vi "example_vector_add_vectors.vi"() -> ()   [LabVIEW 2020]
uses:
  src/vectorstore/abstract_vector_base/abstract_vector_base.lvclass
  src/vectorstore/abstract_vector_base/vector.ctl
  src/models/llm_openai_embedding/llm_openai_embedding.lvclass
  D:/Personal/LabVIEW LLMs/src/models/abstract_llm_base/abstract_llm_base.lvclass
  src/vectorstore/vector_qdrant/vector_qdrant.lvclass
  D:/Personal/LabVIEW LLMs/src/vectorstore/abstract_vector_base/abstract_vector_base.lvclass
  src/models/message_text/message_text.lvclass
  D:/Personal/LabVIEW LLMs/src/models/abstract_message_base/abstract_message_base.lvclass
  src/models/message_vectors/message_vectors.lvclass
  src/models/message_text/create_text_message.vi
  src/models/llm_openai_embedding/Instantiate_llm_openai_embed.vi
  src/models/message_text/get_text_message_value.vi
  src/models/message_vectors/get_vector_message_value.vi
  src/utilities/env_variables/env_variables.lvlib
  src/models/abstract_llm_embedding/abstract_llm_embedding.lvclass
  D:/Personal/LabVIEW LLMs/src/models/message_text/message_text.lvclass
  D:/Personal/LabVIEW LLMs/src/models/message_vectors/message_vectors.lvclass
panel:
  in  "Database":string[](array[string])=["Apple", "USD", "Mango", "Titanic", "Himalayas", "Papaya", "Barrak Obama", "Drangon Fruit", "Cocnut", "Pacific Ocean", "Banana", "Carrot", "Biscut", "Pokemon", "Cherry", "Mothers day"]
  out "error out":errorcluster
  in  "collection_name":string="my_collection"
  in  "Vector Selector":enum32{"qdrant", "weviate"}(tab)
  in  "host_url":string="http://localhost:6333/"
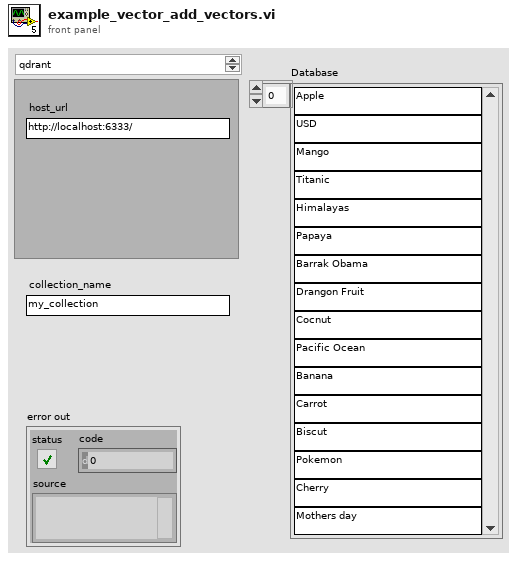
[diagram p1: front panel]
types:
  T1 = typedef "abstract_vector_base.lvclass/vector.ctl" = cluster{"id":string, "vector":dbl[], "text":string, "metadata":cluster{"key":string, "value":string}[]}
  T2 = typedef "message_vectors.lvclass/embedding.ctl" = cluster{"index":u32, "Vectors":dbl[]}
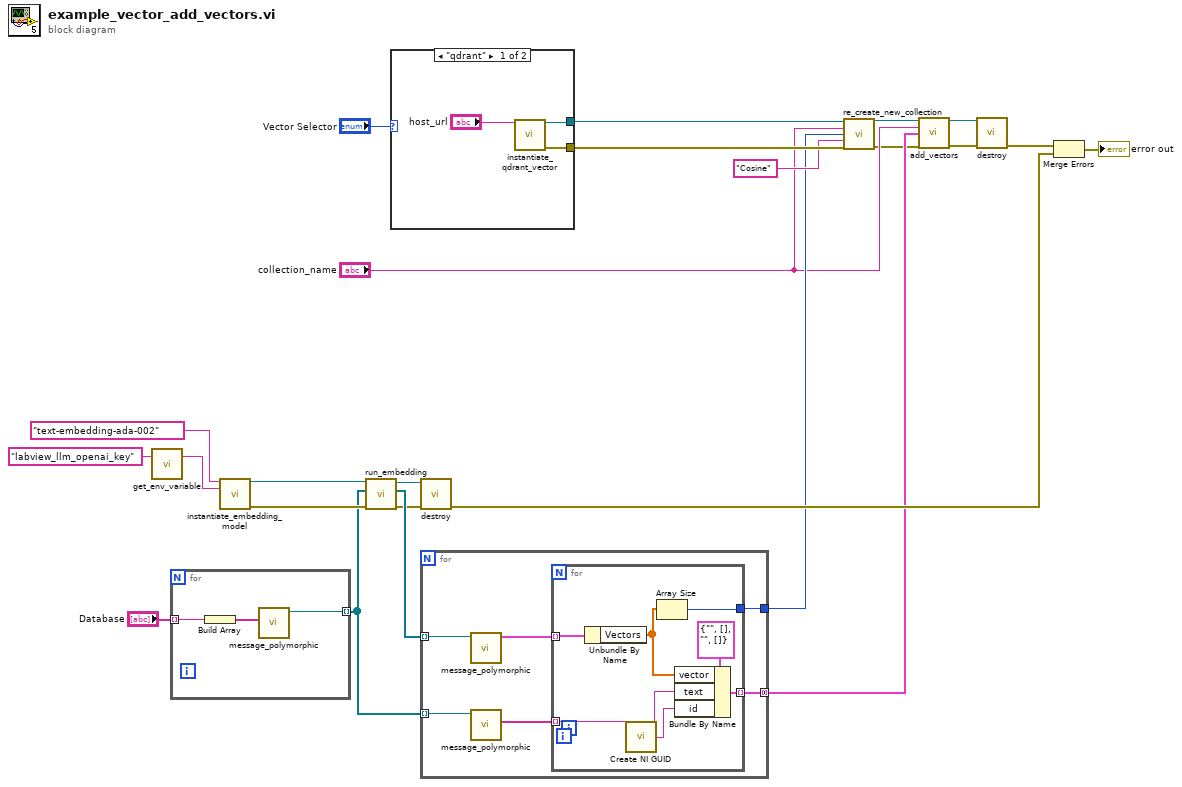
[diagram p0: block diagram]
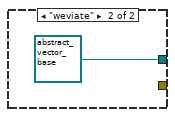
[diagram p2: hidden frame]
diagram:
  n1 = call "get_env_variable.vi"("Environment Variable Name"="labview_llm_openai_key") -> ("Value"=w15:string)  [unwired: 1 in, 1 out]
  n2 = for {
    tunnel: "Database" -> [w27] mode=indexing
    tunnel: [w26] -> w10 mode=indexing
    n3 = Build Array(w27) -> (w25:string[])
    n4 = call-poly "message_polymorphic.vi"("content"=w25) -> ("message_text out"=w26:refnum<class "message_text.lvclass">)  [unwired: 9 in, 1 out]
  }
  n5 = call-poly "instantiate_embedding_model.vi"("model_name"="text-embedding-ada-002", "openai_key"=w15) -> ("llm_openai_embedding out"=w17:refnum<class "llm_openai_embedding.lvclass">, "error out"=w18:errorcluster)  [unwired: 12 in]
  n6 = call "run_embedding.vi"("error in (no error)"=w18, "Messages"=w10, "abstract_llm_embedding in"=w17) -> ("error out"=w6:errorcluster, "Response"=w19:refnum<class "message_vectors.lvclass">[], "abstract_llm_embedding out"=w7:refnum<class "llm_openai_embedding.lvclass">)  [unwired: 6 in]
  n7 = case shown="\"qdrant\"" "Vector Selector" {
    tunnel: [w30 refnum<class "abstract_vector_base.lvclass"> refnum ("abstract_vector_base.lvclass")] -> w22
    tunnel: [w28 _] -> w21
    frame "qdrant" {
      n8 = call "instantiate_qdrant_vector.vi"("host_url"="host_url") -> ("vector_qdrant out"=w30:refnum<class "vector_qdrant.lvclass">, "error out"=w28:errorcluster)  [unwired: 13 in]
    }
    frame "weviate" {
    }
  }
  n9 = call-dynamic "destroy.vi"("error in (no error)"=w6, "llm_openai_embedding in"=w7) -> ("error out"=w11:errorcluster)  [unwired: 8 in, 1 out]
  n10 = for {
    tunnel: w19 -> [w37] mode=indexing
    tunnel: w10 -> [w36] mode=indexing
    tunnel: [w33] -> w8 mode=concatenating
    tunnel: [w32] -> w9
    n11 = call-poly "message_polymorphic.vi"("message_vectors in"=w37) -> ("embedding_data"=w35:T2[])  [unwired: 9 in, 1 out]
    n12 = call-poly "message_polymorphic.vi"("abstract_message_base.lvclass"=w36) -> ("content"=w34:string[])  [unwired: 8 in, 2 out]
    n13 = for {
      tunnel: w35 -> [w43] mode=indexing
      tunnel: w34 -> [w42] mode=indexing
      tunnel: [w41] -> w33 mode=indexing
      tunnel: [w38] -> w32
      n14 = Unbundle By Name(w43) -> ("Vectors"=w40:dbl[])
      n15 = call <vilib>:"Create NI GUID.vi"() -> ("NI GUID"=w39:string)
      n16 = Array Size(array=w40) -> (size(s)=w38:i32)
      n17 = Bundle By Name(cluster=T1 {"id"="", "vector"=[], "text"="", "metadata"=[]} ("vector"), "vector"=w40, "text"=w42, "id"=w39) -> (w41:T1)
    }
  }
  n18 = call-dynamic "re_create_new_collection.vi"("abstract_vector_base in"=w22, "collection_name"="collection_name", "vector_size"=w9, "distance"="Cosine", "error in (no error)"=w21) -> ("abstract_vector_base out"=w2:refnum<class "abstract_vector_base.lvclass">, "error out"=w3:errorcluster)  [unwired: 9 in]
  n19 = call-dynamic "add_vectors.vi"("abstract_vector_base in"=w2, "colection_name"="collection_name", "vectors"=w8, "error in (no error)"=w3) -> ("abstract_vector_base out"=w5:refnum<class "abstract_vector_base.lvclass">, "error out"=w1:errorcluster)  [unwired: 10 in]
  n20 = call-dynamic "destroy.vi"("abstract_vector_base in"=w5, "error in (no error)"=w1) -> ("error out"=w23:errorcluster)  [unwired: 12 in, 1 out]
  n21 = Merge Errors(w23, w11) -> (→"error out":errorcluster)
